vi "niSE Connect.vi"(6 "wait_for_rebounce":bool, 7 "multi_connect_mode":T1, 8 "error in (no error)":errorcluster, 10 "connection_specification":string, 11 "Session Factory in":refnum<class "Session Factory.lvclass">) -> (0 "error out":errorcluster, 3 "Session Factory out":refnum<class "Session Factory.lvclass">)   [LabVIEW 2021, in "NI Session Management niSE.lvlib" / "Session Factory.lvclass"]
uses:
  Session Factory.lvclass
  basic_switch_executive_driver_client/RPC Messages/nise_MulticonnectMode.ctl
  basic_switch_executive_driver_client/RPC Messages/nise_ConnectInfo.ctl
  basic_switch_executive_driver_client/RPC Messages/nise_SessionInformation.ctl
  <vilib>/Plug-In SDKs/Clients/Session Management V1/Session Reservation/Initialize and Close Session Behavior.ctl
  Session Factory.lvclass/Session Factory.ctl
  basic_switch_executive_driver_client/basic_switch_executive_driver_client.lvlib
  <vilib>/Plug-In SDKs/Clients/Session Management V1/Session Reservation/Session Reservation.lvclass
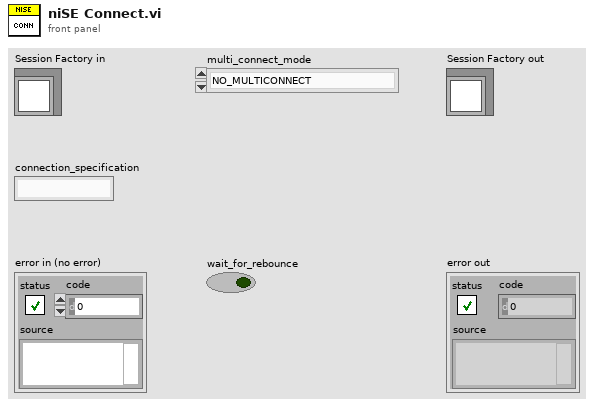
[diagram p1: front panel]
types:
  T1 = typedef "basic_switch_executive_driver_client.lvlib/nise_MulticonnectMode.ctl" = enum32{"NO_MULTICONNECT", "USE_DEFAULT_MODE", "MULTICONNECT_ROUTES"}
  T2 = typedef "basic_switch_executive_driver_client.lvlib/nise_ConnectInfo.ctl" = cluster{"connection_specification":string, "session_info":T3, "wait_for_rebounce":bool, "multi_connect_mode":T1}
  T3 = typedef "basic_switch_executive_driver_client.lvlib/nise_SessionInformation.ctl" = cluster{"session_id":u32, "initialize_and_close_session_behavior":T4}
  T4 = typedef "NI Session Management V1 Client.lvlib/Session Reservation.lvclass/Initialize and Close Session Behavior.ctl" = enum16{"Auto", "Initialize and Close", "Attach and Detach", "Initialize and Detach", "Attach and Close"}
  T5 = typedef "grpc-lvsupport-release.lvlib/grpcId.ctl" = u64
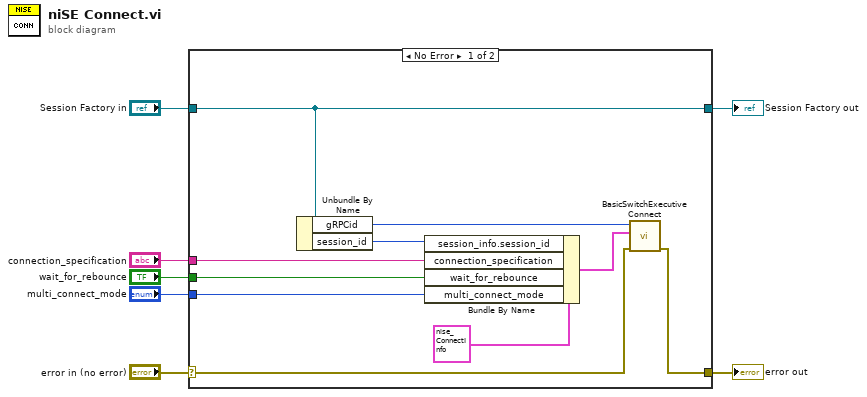
[diagram p0: block diagram]
diagram:
  n1 = case shown="No Error" "error in (no error)" {
    selector: "error in (no error)" -> [w13 w19]
    tunnel: [w12 w19] -> w6
    tunnel: [w17 w18] -> w4
    tunnel: "Session Factory in" -> [w17 w18]
    tunnel: "connection_specification" -> [w11 _]
    tunnel: "wait_for_rebounce" -> [w9 _]
    tunnel: "multi_connect_mode" -> [w8 _]
    frame No Error {
      n2 = Unbundle By Name(w17) -> ("gRPCid"=w16:T5, "session_id"=w10:u32)
      n3 = Bundle By Name(cluster=T2 {"connection_specification"="", "session_info"={"session_id"=0, "initialize_and_close_session_behavior"=enum."Auto"}, "wait_for_rebounce"=FALSE, "multi_connect_mode"=enum."NO_MULTICONNECT"} ("Request Data"), "session_info.session_id"=w10, "connection_specification"=w11, "wait_for_rebounce"=w9, "multi_connect_mode"=w8) -> (w14:T2)
      n4 = call "BasicSwitchExecutive Connect.vi"("error in"=w13, "Request Data"=w14, "gRPC ID"=w16) -> ("error out"=w12:errorcluster)  [unwired: 6 in, 2 out]
    }
    frame Error {
    }
  }
  "error out" <- w6
  "Session Factory out" <- w4
